vi "get_target_pos_by_name.vi"(8 "error in (no error)":errorcluster caption="错误输入（无错误）", 9 "name":string, 10 "target pos with offset":dbl, 11 "MotorSystem 输入":refnum<class "MotorSystem.lvclass">) -> (0 "error out":errorcluster caption="错误输出", 2 "target pos":dbl, 3 "MotorSystem 输出":refnum<class "MotorSystem.lvclass">)   [LabVIEW 2016, in "MotionControl_UFO_3DOF.lvlib" / "MotorSystem.lvclass"]
uses:
  <userlib>/MotionControl_UFO_3DOF/MotorSystem/MotorSystem.lvclass
  <userlib>/MotionControl_UFO_3DOF/MotorSystem/MotorSystem.lvclass/MotorSystem.ctl
  <userlib>/MotionControl_UFO_3DOF/OneMotion/OneMotion.lvclass/OneMotion.ctl
  <userlib>/MotionControl_UFO_3DOF/OneMotion/OneMotion.lvclass
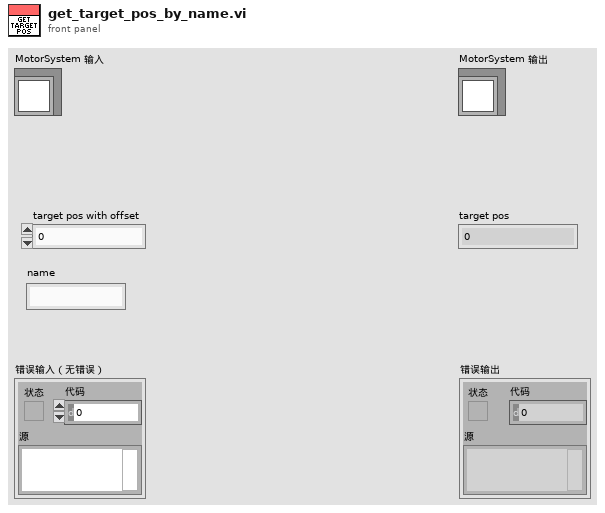
[diagram p1: front panel]
types:
  T1 = typedef "MotionControl_UFO_3DOF.lvlib/MotorSystem.lvclass/MotionCluster.ctl" = cluster{"OneMotion.lvclass":refnum<class "OneMotion.lvclass">, "connected?":bool, "default enabled?":bool, "enabled?":bool}
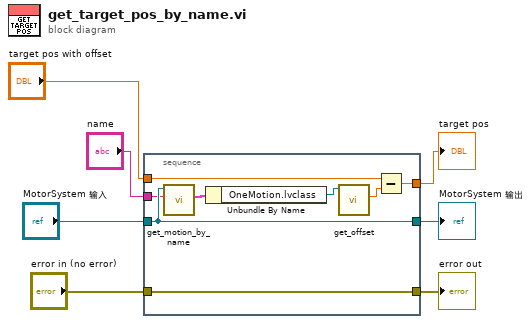
[diagram p0: block diagram]
diagram:
  n1 = stacked-sequence {
    tunnel: [w15] -> w7
    tunnel: [w14] -> w5
    tunnel: "MotorSystem 输入" -> [w14]
    tunnel: "error in (no error)" -> [w15]
    tunnel: "name" -> [w13]
    tunnel: "target pos with offset" -> [w10]
    tunnel: [w8] -> w1
    frame #0 {
      n2 = call <userlib>:"get_motion_by_name.vi"("name"=w13, "MotorSystem in"=w14) -> ("motion cluster"=w12:T1)  [unwired: 7 in, 2 out]
      n3 = Unbundle By Name(w12) -> ("OneMotion.lvclass"=w11:refnum<class "OneMotion.lvclass">)
      n4 = call <userlib>:"get_offset.vi"("OneMotion输入"=w11) -> ("offset"=w9:dbl)  [unwired: 8 in, 2 out]
      n5 = Subtract(x=w10, y=w9) -> (x-y=w8:dbl)
    }
  }
  "error out" <- w7
  "MotorSystem 输出" <- w5
  "target pos" <- w1
